vi "Write Logged Data.vi"(8 "error in (no error)":errorcluster, 10 "Data":T1[](array[typedef]), 11 "CSV Word Logger in":refnum<class "CSV Word Logger.lvclass">) -> (0 "error out":errorcluster, 3 "CSV Word Logger out":refnum<class "CSV Word Logger.lvclass">)   [LabVIEW 2020, in "AIM ARINC 429 Engine.lvlib" / "Implementation.lvlib" / "CSV Word Logger.lvclass"]
uses:
  CSV Word Logger.lvclass
  3e68417c-88ea-46f3-a078-ba49f2c6225d.vi
  Word.ctl
  Implementation.lvlib
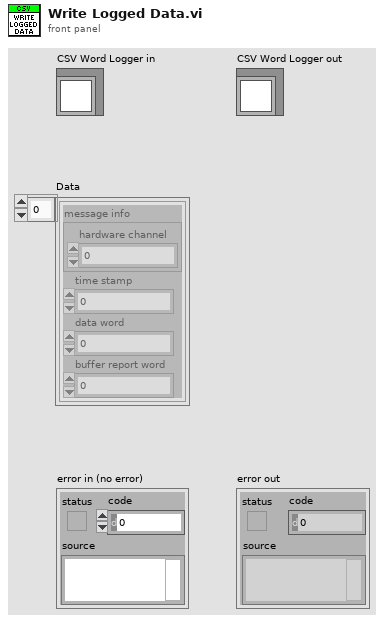
[diagram p1: front panel]
types:
  T1 = typedef "AIM ARINC 429 Engine.lvlib/Implementation.lvlib/Word.ctl" = cluster{"message info":cluster{"hardware channel":u8}, "time stamp":dbl, "data word":u32, "buffer report word":u32}
  T2 = typedef "Data Word Format.ctl" = string
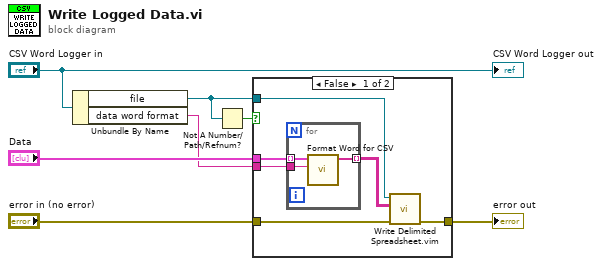
[diagram p0: block diagram]
diagram:
  n1 = Unbundle By Name("CSV Word Logger in") -> ("file"=w3:refnum<file>, "data word format"=w1:T2)
  n2 = Not A Number/Path/Refnum?(number/path/refnum=w3) -> (NaN/Path/Refnum?=w2:bool)
  n3 = case shown="False" w2 {
    tunnel: "Data" -> [w13 _]
    tunnel: w3 -> [w11 _]
    tunnel: "error in (no error)" -> [w10 w17]
    tunnel: [w9 w17] -> w4
    tunnel: w1 -> [w8 _]
    frame False {
      n4 = for {
        tunnel: w13 -> [w16] mode=indexing
        tunnel: [w15] -> w12 mode=indexing
        tunnel: w8 -> [w14]
        n5 = call "Format Word for CSV.vi"("Data Word Format"=w14, "word"=w16) -> ("string array"=w15:string[])  [unwired: 9 in]
      }
      n6 = call "Write Delimited Spreadsheet.vim"("error in (no error)"=w10, "data"=w12, "file in"=w11) -> ("error out"=w9:errorcluster)  [unwired: 7 in, 1 out]
    }
    frame True {
    }
  }
  "error out" <- w4
  "CSV Word Logger out" <- "CSV Word Logger in"
